vi "Pattern ROI (SubVI).vi"(6 "divider":sgl, 9 "number of matches":bool, 10 "Calibrated Matches (Geometric Matching 1)":T1[](array[typedef]) {"Correlation Score" format="%.2f"; "Target Template Curve Score" format="%.2f"; "Template Target Curve Score" format="%.2f"; "Bounding Box"."y" format="%.2f"; "Bounding Box"."x" format="%.2f"; "Position"."y" format="%.2f"; "Position"."x" format="%.2f"; "Score" format="%.2f"; "Scale" format="%.2f"; "Angle" format="%.2f"; "Occlusion %" format="%.2f"}, 11 "Contours in":T2(array[cluster])) -> (1 "y1":i32, 2 "x1":i32, 3 "y0":i32, 4 "Scale":sgl, 5 "x0":i32, 7 "Contours out":T2(array[cluster]))   [LabVIEW 2017]
uses:
  <vilib>/vision/Pattern Matching.llb/IMAQ GM Match Report.ctl
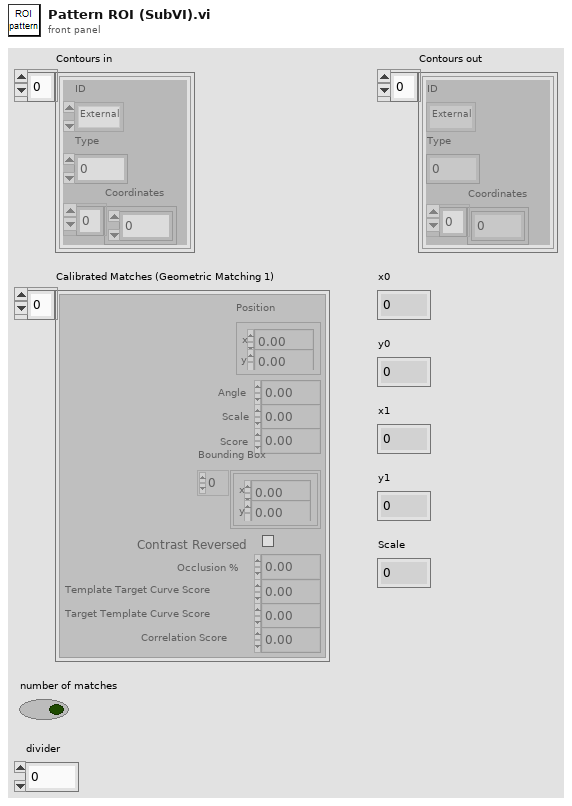
[diagram p1: front panel]
types:
  T1 = typedef "IMAQ GM Match Report.ctl" = cluster{"Position":cluster{"x":sgl, "y":sgl}, "Angle":sgl, "Scale":sgl, "Score":sgl, "Bounding Box":cluster{"x":sgl, "y":sgl}[], "Contrast Reversed":bool, "Occlusion %":sgl, "Template Target Curve Score":sgl, "Target Template Curve Score":sgl, "Correlation Score":sgl}
  T2 = cluster{"ID":enum32{"External", "Internal"}, "Type":u32, "Coordinates":i32[]}[]
  T3 = cluster{"ID":enum32{"External", "Internal"}, "Type":u32, "Coordinates":i32[]}
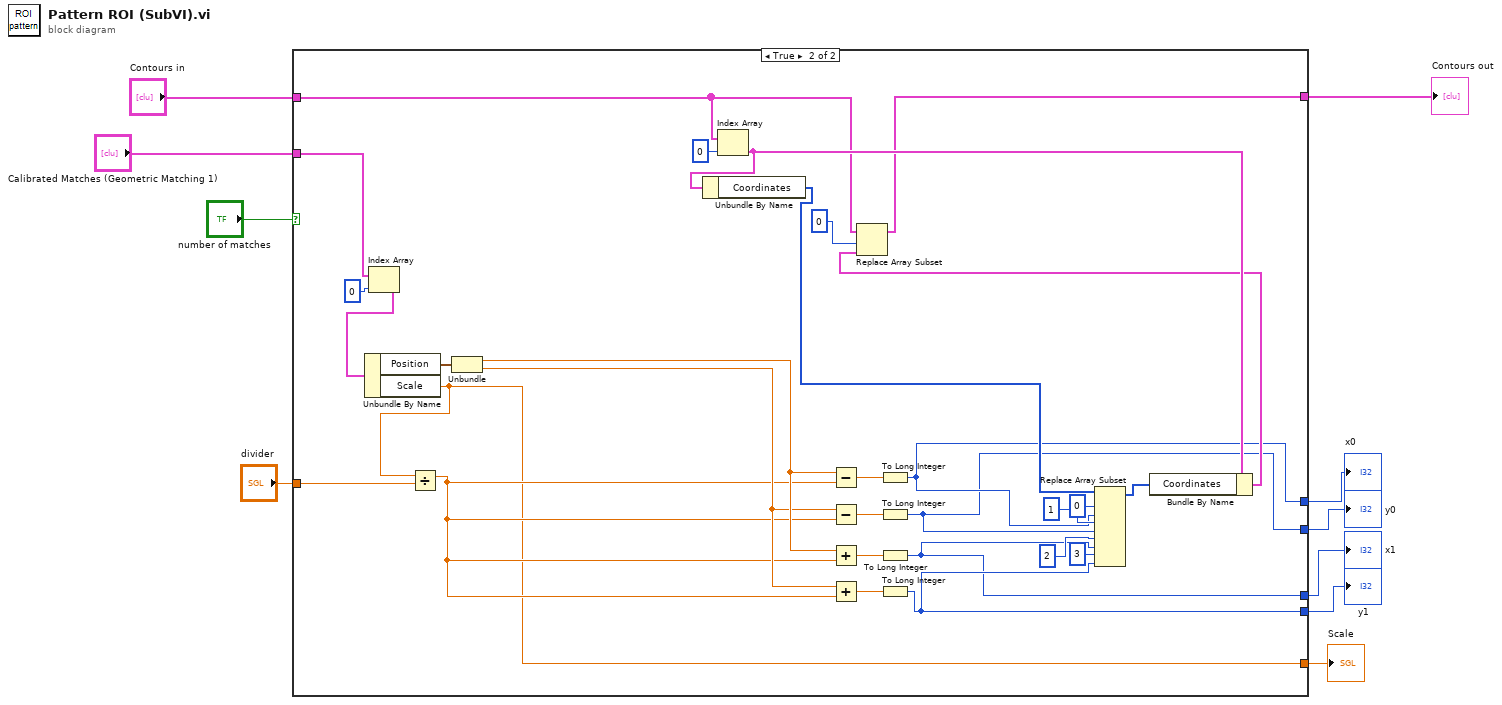
[diagram p0: block diagram]
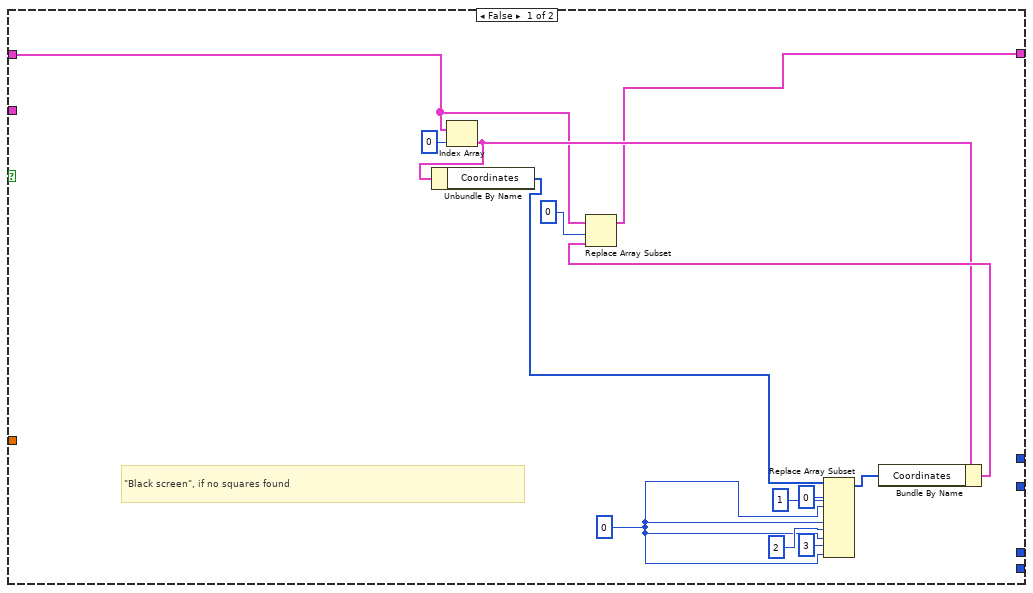
[diagram p2: hidden frame]
diagram:
  n1 = case shown="True" "number of matches" {
    tunnel: "Calibrated Matches (Geometric Matching 1)" -> [_ w32]
    tunnel: [_ w31] -> w3
    tunnel: "divider" -> [_ w30]
    tunnel: [_ w29] -> w5
    tunnel: [_ w28] -> w6
    tunnel: [_ w27] -> w7
    tunnel: [_ w26] -> w8
    tunnel: "Contours in" -> [w11 w25]
    tunnel: [w12 w24] -> w10
    frame False {
      w13 = 0 ("index")
      # "\"Black screen\", if no squares found"
      n2 = Index Array(array=w11, index=0) -> (element=w21:T3)
      n3 = Unbundle By Name(w21) -> ("Coordinates"=w20:i32[])
      n4 = Replace Array Subset(array=w20, new element #1=w13, index #1=0 ("index"), new element #2=w13, index #2=1 ("index"), new element #3=w13, index #3=2 ("index"), new element #4=w13, index #4=3 ("index")) -> (w22:i32[])
      n5 = Bundle By Name(cluster=w21, "Coordinates"=w22) -> (w23:T3)
      n6 = Replace Array Subset(array=w11, new element=w23, index=0) -> (w12:T2)
    }
    frame True {
      n7 = Index Array(array=w32, index=0) -> (element=w51:T1)
      n8 = Unbundle By Name(w51) -> ("Position"=w50:cluster{"x":sgl, "y":sgl}, "Scale"=w31:sgl)
      n9 = Divide(x=w31, y=w30) -> (x/y=w33:sgl)
      n10 = Unbundle(w50) -> ("x"=w47:sgl, "y"=w46:sgl)
      n11 = Index Array(array=w25, index=0) -> (element=w39:T3)
      n12 = Unbundle By Name(w39) -> ("Coordinates"=w41:i32[])
      n13 = Subtract(x=w47, y=w33) -> (x-y=w45:sgl)
      n14 = Subtract(x=w46, y=w33) -> (x-y=w44:sgl)
      n15 = Add(x=w47, y=w33) -> (x+y=w42:sgl)
      n16 = Add(x=w46, y=w33) -> (x+y=w43:sgl)
      n17 = To Long Integer(number=w45) -> (32bit integer=w27:i32)
      n18 = To Long Integer(number=w44) -> (32bit integer=w26:i32)
      n19 = To Long Integer(number=w42) -> (32bit integer=w28:i32)
      n20 = To Long Integer(number=w43) -> (32bit integer=w29:i32)
      n21 = Replace Array Subset(array=w41, new element #1=w27, index #1=0 ("index"), new element #2=w26, index #2=1 ("index"), new element #3=w28, index #3=2 ("index"), new element #4=w29, index #4=3 ("index")) -> (w38:i32[])
      n22 = Bundle By Name(cluster=w39, "Coordinates"=w38) -> (w37:T3)
      n23 = Replace Array Subset(array=w25, new element=w37, index=0) -> (w24:T2)
    }
  }
  "Contours out" <- w10
  "y0" <- w8
  "x0" <- w7
  "x1" <- w6
  "y1" <- w5
  "Scale" <- w3
